vi "下载方式.vi"() -> (3 "下载方式":enum32{"数据线", "WIFI", "取消"}(ring))   [LabVIEW 2018]
panel:
  in  "取消":bool
  in  "确认":bool
  in  "单选按钮":enum32{"数据线", "WIFI", "取消"}(radio)
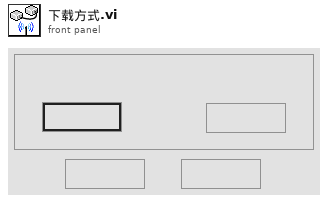
[diagram p1: front panel]
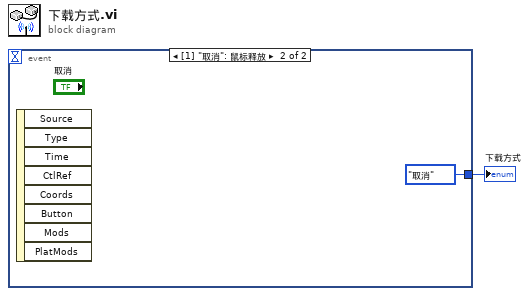
[diagram p0: block diagram]
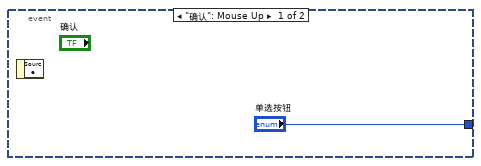
[diagram p2: hidden frame]
diagram:
  n1 = event shown="[1] \"取消\": 鼠标释放" {
    selector: _ -> [_ _]
    dyn-events: _ -> [_ _]
    timeout: _ -> [_ _]
    tunnel: ["单选按钮" enum32{"数据线", "WIFI", "取消"}."取消" ("单选按钮")] -> w1
    event "确认": Mouse Up {
      n2 = event-data() -> ()  [unwired: 1 in, 1 out]
    }
    event "取消": Mouse Up {
      n3 = event-data() -> ()  [unwired: 1 in, 8 out]
    }
  }
  "下载方式" <- w1
